vi "dmm_configure_volts.vi"(4 "Sequence Context":T1) -> (0 "error out":errorcluster, 1 "Test Data":T2 {"Numeric Measurement" format="%.2f"})   [LabVIEW 2012]
uses:
  <vilib>/addons/TestStand/_TSUtility.llb/TestStand - Get Property Value (String).vi
  Demo/LabVIEW/SupportVIs.llb/LabVIEW Test - Test Data.ctl
  <vilib>/addons/TestStand/_TSLegacy.llb/LabVIEW Test - Sequence Context.ctl
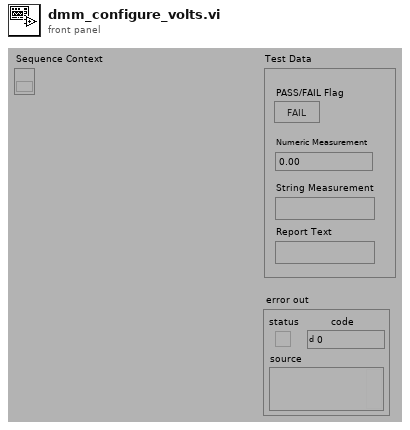
[diagram p1: front panel]
types:
  T1 = typedef "LabVIEW Test - Sequence Context.ctl" = refnum<k7>
  T2 = typedef "LabVIEW Test - Test Data.ctl" = cluster{"PASS/FAIL Flag":bool, "Numeric Measurement":dbl, "String Measurement":string, "Report Text":string}
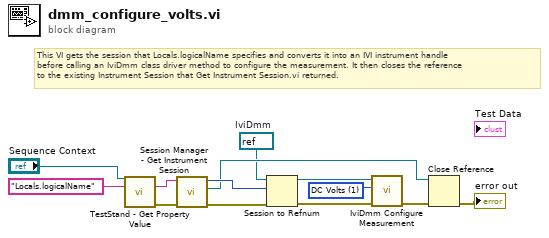
[diagram p0: block diagram]
diagram:
  w1 = refnum<k15> refnum  # IviDmm
  w5 = 1 items=["DC Volts"=1, "AC Volts"=2, "DC Current"=3, "AC Current"=4, "2 Wire Resistance"=5, "4 Wire Resistance"=101, "AC + DC Volts"=106, "AC + DC Current"=107, "Frequency"=104, "Period"=105, "Temperature"=108] ("measurement function (DC Volts)")
  # "This VI gets the session that Locals.logicalName specifies and converts it into an IVI instrument handle\nbefore calling an IviDmm class driver method to configure the measurement. It then closes the reference\nto the existing Instrument Session that Get Instrument Session.vi returned."
  n1 = call-poly <vilib>:"TestStand - Get Property Value.vi"("Sequence Context In"="Sequence Context", "Lookup String"="Locals.logicalName") -> ("Value"=w8:string, "error out"=w7:errorcluster)  [unwired: 1 in, 11 out]
  n2 = call <vilib>:"Session Manager - Get Instrument Session.vi"("error in (no error)"=w7, "Session Name"=w8) -> ("error out"=w12:errorcluster, "Instrument Session"=w3:refnum<k7>, "Driver Handle"=w13:u32)  [unwired: 1 in, 6 out]
  n3 = Session to Refnum(4:w12, 6:w13, 7:w1) -> (0:w11:errorcluster, 3:w10:refnum<k15>)
  n4 = call <vilib>:"IviDmm Configure Measurement.vi"("error in (no error)"=w11, "measurement function (DC Volts)"=w5, "instrument handle"=w10) -> ("error out"=w4:errorcluster)  [unwired: 2 in, 6 out]
  n5 = Close Reference(reference=w3, error in (no error)=w4) -> (error out=→"error out":errorcluster)
